vi "load config data.vi"(8 "error in (no error)":errorcluster, 11 "Base in":refnum<class "Base.lvclass">) -> (0 "error out":errorcluster, 3 "Base out":refnum<class "Base.lvclass">)   [LabVIEW 2022 SP3, in "Base.lvclass"]
uses:
  Base.lvclass
  Base.lvclass/Base.ctl
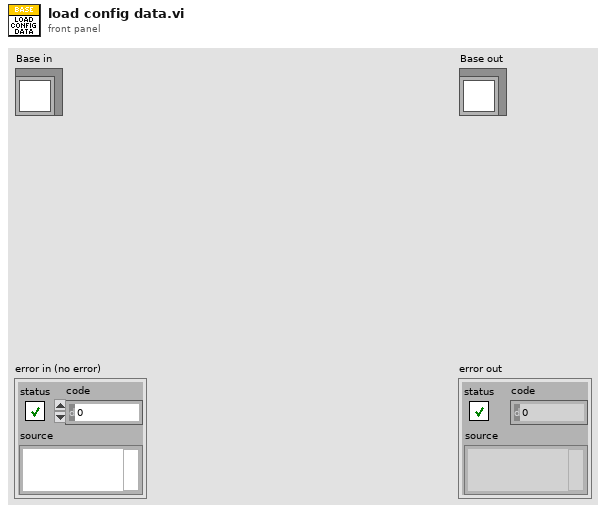
[diagram p1: front panel]
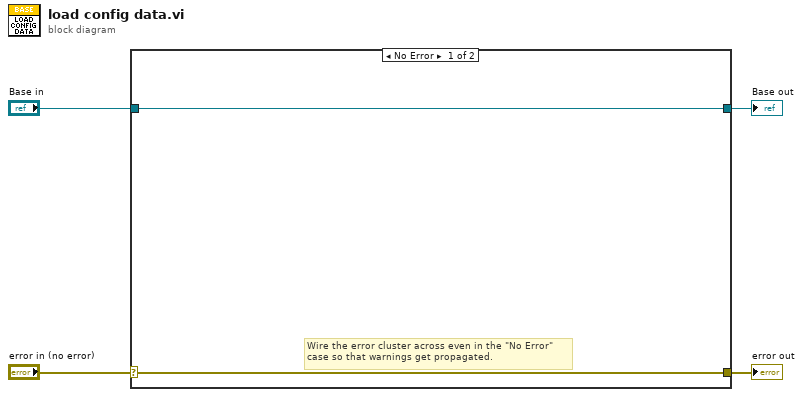
[diagram p0: block diagram]
diagram:
  n1 = case shown="No Error" "error in (no error)" {
    selector: "error in (no error)" -> [w5 w8]
    tunnel: [w5 w8] -> w3
    tunnel: [w6 w7] -> w1
    tunnel: "Base in" -> [w6 w7]
    frame No Error {
      # "Wire the error cluster across even in the \"No Error\"\ncase so that warnings get propagated."
    }
    frame Error {
    }
  }
  "error out" <- w3
  "Base out" <- w1
